vi "isResponseAvailable.vi"(8 "error in (no error)":errorcluster, 9 "Function":u8, 10 "Address":u8, 11 "Mockbus in":refnum<class "Mockbus.lvclass">) -> (0 "error out":errorcluster, 2 "Available?":bool, 3 "Mockbus out":refnum<class "Mockbus.lvclass">)   [LabVIEW 2015, in "Mockbus.lvclass"]
uses:
  Mockbus.lvclass
  Mockbus.lvclass/Mockbus.ctl
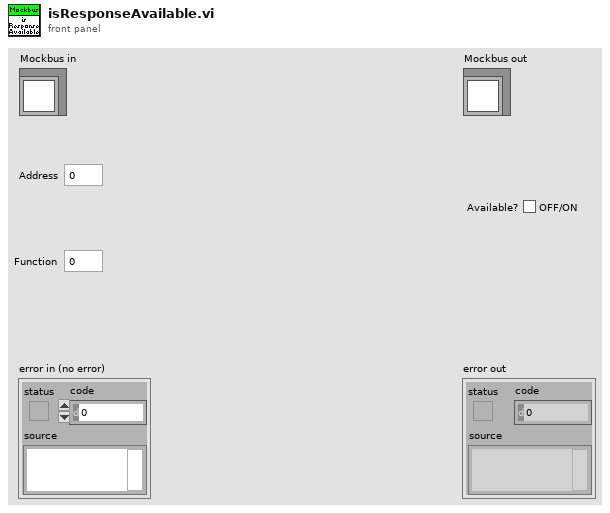
[diagram p1: front panel]
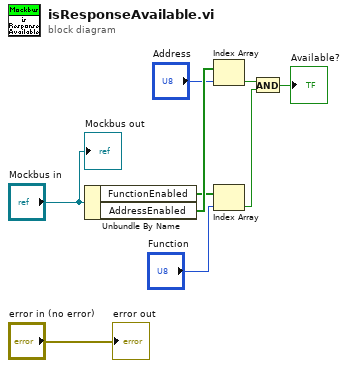
[diagram p0: block diagram]
diagram:
  n1 = Unbundle By Name("Mockbus in") -> ("FunctionEnabled"=w7:bool[], "AddressEnabled"=w9:bool[])
  n2 = Index Array(array=w9, index="Address") -> (element=w4:bool)
  n3 = Index Array(array=w7, index="Function") -> (element=w5:bool)
  n4 = And(x=w4, y=w5) -> (x .and. y?=→"Available?":bool)
  "error out" <- "error in (no error)"
  "Mockbus out" <- "Mockbus in"
